vi "run.vi"(8 "error in (no error)":errorcluster, 11 "ImagingModeDL090130Frame in":refnum<class "ImagingModeDL090130Frame.lvclass">=refnum) -> (0 "error out":errorcluster, 3 "ImagingModeDL090130Frame out":refnum<class "ImagingModeDL090130Frame.lvclass">)   [LabVIEW 2010, in "ImagingModeDL090130Frame.lvclass"]
uses:
  ImagingModeDL090130Frame.lvclass
  internal_trigger_enum.ctl
  main/labview_source/controls/undock_button.ctl
  translation_mode_enum.ctl
  common/xcontrols/XSettings/XSettings/XSettings.xctl
  common/classes/GenericComponent/GenericComponent/GenericComponent.lvclass
  common/xcontrols/XIntensityCompensation/XIntensityCompensation/XIntensityCompensation.xctl
  speed_constant_enum.ctl
  control_refs.ctl
  state_enum.ctl
  common/classes/GenericToplevelComponent/GenericToplevelComponent/trigger_type_enum.ctl
  GenericImagingMode/GenericImagingMode/GenericImagingMode.lvclass
  ImagingModeDL090130Frame.lvclass/ImagingModeDL090130Frame.ctl
  Trajectory/GenericTrajectory/GenericTrajectory/GenericTrajectory.lvclass
  common/classes/ErrorController/ErrorController/class_data.vi
  common/classes/ErrorController/ErrorController/ErrorController.lvclass
panel:
  out "settings enforced?":bool
  in  "button:undock":T1
  in  "Tab Control":enum32{"User", "Debug", "About"}(tab)
  in  "XIntensityCompensation":cluster{"A":dbl, "lambda":dbl[unit], "C":dbl}(xcontrol)
  in  "translation mode":T2
  in  "return to origin?":bool=TRUE
  in  "step":dbl[unit] min=0.0 max=0.01 step=1e-07
  in  "no. of averagings":i32=1 caption="averaging" min=1 max=100
  in  "movie duration":dbl[unit]=10.24 min=0.0 max=3600.0
  in  "no. of frames":i32=20 caption="frames" min=1 max=100000
  in  "defineButton":bool
  in  "frame rate":dbl[unit]=1.953125 min=0.0 max=100.0
  in  "pixel dwell time":dbl[unit]=7.8125e-06 min=0.0 max=0.001
  in  "line scan time":dbl[unit]=0.002 min=0.0 max=1.0
  in  "y aspect":dbl=1.0 caption=":" min=0.0
  in  "x aspect":dbl=1.0 caption="aspect ratio (x:y)" min=0.0 step=1.0
  in  "y lines":i32=256 min=0 max=1000
  out "offset":dbl[unit]
  in  "x pixels":i32=256 min=0 max=1000 step=1
  out "frame no.":i32=12 caption="frame"
  out "repetition no.":i32=1 caption="repetition"
  in  "settings":refnum<class "GenericComponent.lvclass">(xcontrol)
  in  "keep constant":T3
  out "event handling loop counter":i32=10
  out "statemachine loop counter":i32=75
  out "event error":errorcluster
  out "action handler error":errorcluster
  out "finished?":bool
  out "last trigger":T4
  out "internal triggers":T4[](array[typedef])
  # "stack settings"
  # "frame settings"
  # "current values"
  # "ImagingModeDL090130Frame"
  # "Implemented by: \nDominik Langer, University of Zurich"
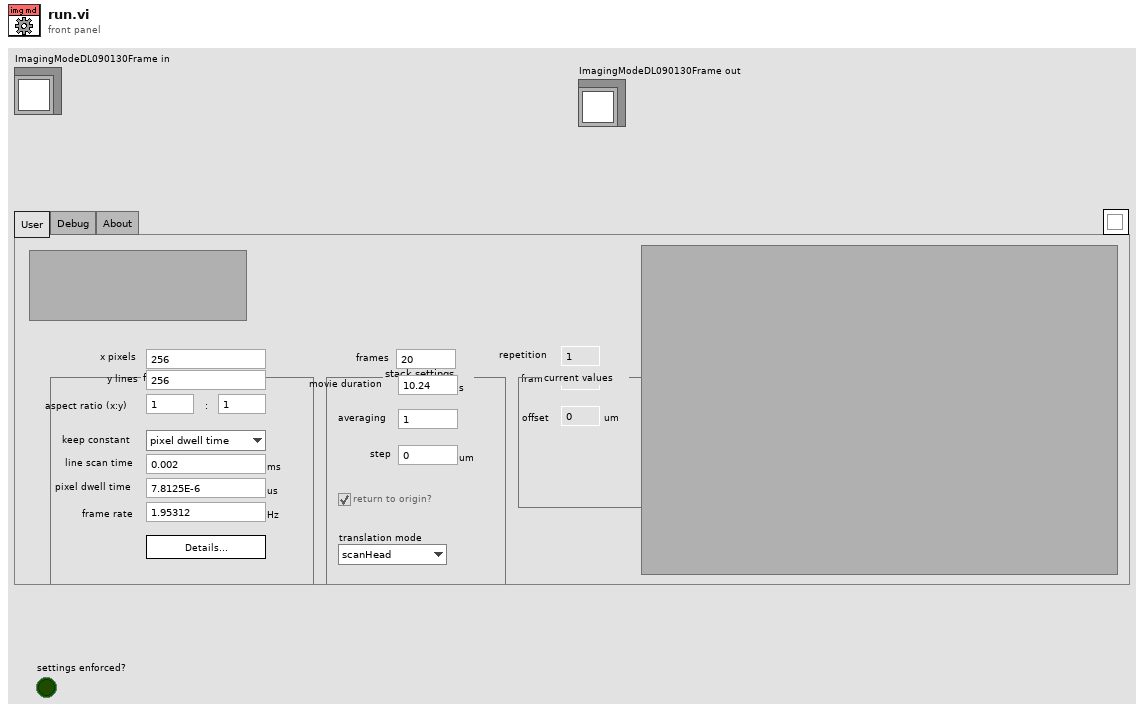
[diagram p1: front panel]
types:
  T1 = typedef "undock_button.ctl" = bool
  T2 = typedef "ImagingModeDL090130Frame.lvclass/translation_mode_enum.ctl" = enum16{"scanHead", "stage"}
  T3 = typedef "ImagingModeDL090130Frame.lvclass/speed_constant_enum.ctl" = enum16{"pixel dwell time", "line scan time", "frame rate"}
  T4 = typedef "ImagingModeDL090130Frame.lvclass/internal_trigger_enum.ctl" = enum16{"NULL", "initialise", "terminate", "start", "stop", "proceed", "update", "translate", "start scanning"}
  T5 = typedef "ImagingModeDL090130Frame.lvclass/control_refs.ctl" = cluster{"resolution controls":cluster{"x pixels":refnum<vi>, "y pixels":refnum<vi>, "ratio x factor":refnum<vi>, "ratio y factor":refnum<vi>}, "speed controls":cluster{"pixel dwell time":refnum<vi>, "line scan time":refnum<vi>, "frame rate":refnum<vi>, "keep constant":refnum<vi>}, "number of frames controls":cluster{"# of frames":refnum<vi>, "duration":refnum<vi>, "# of repetitions":refnum<vi>}, "current value indicators":cluster{"frame #":refnum<vi>, "repetition #":refnum<vi>, "offset":refnum<vi>}, "step controls":cluster{"step size":refnum<vi>, "return to origin?":refnum<vi>, "translation mode":refnum<vi>, "XIntensityCompensation":refnum<vi>}, "settings":refnum<vi>, "defineButton":refnum<vi>, "settings enforced?":refnum<vi>}
  T6 = typedef "ImagingModeDL090130Frame.lvclass/state_enum.ctl" = enum16{"idle", "sweep (scanning)", "sweep (translating)"}
  T7 = typedef "trigger_type_enum.ctl" = enum8{"external", "internal", "common"}
  T8 = typedef "main_trigger_enum.ctl" = enum16{"NULL", "initialise", "terminate", "start", "stop", "change objective", "change experimentController", "change imagingMode", "save notebook", "started saving", "finished saving", "expCtr ready", "expCtr missing", "imgMd ready", "imgMd missing", "scanHd ready", "scanHd missing", "DAQ ready", "DAQ missing", "imgAsm ready", "imgAsm missing", "dataColl ready", "dataColl missing", "display ready", "display missing", "analysr ready", "analysr missing", "instrmnt ready", "instrmnt missing", "stimltr ready", "stimltr missing", "stage ready", "stage missing"}
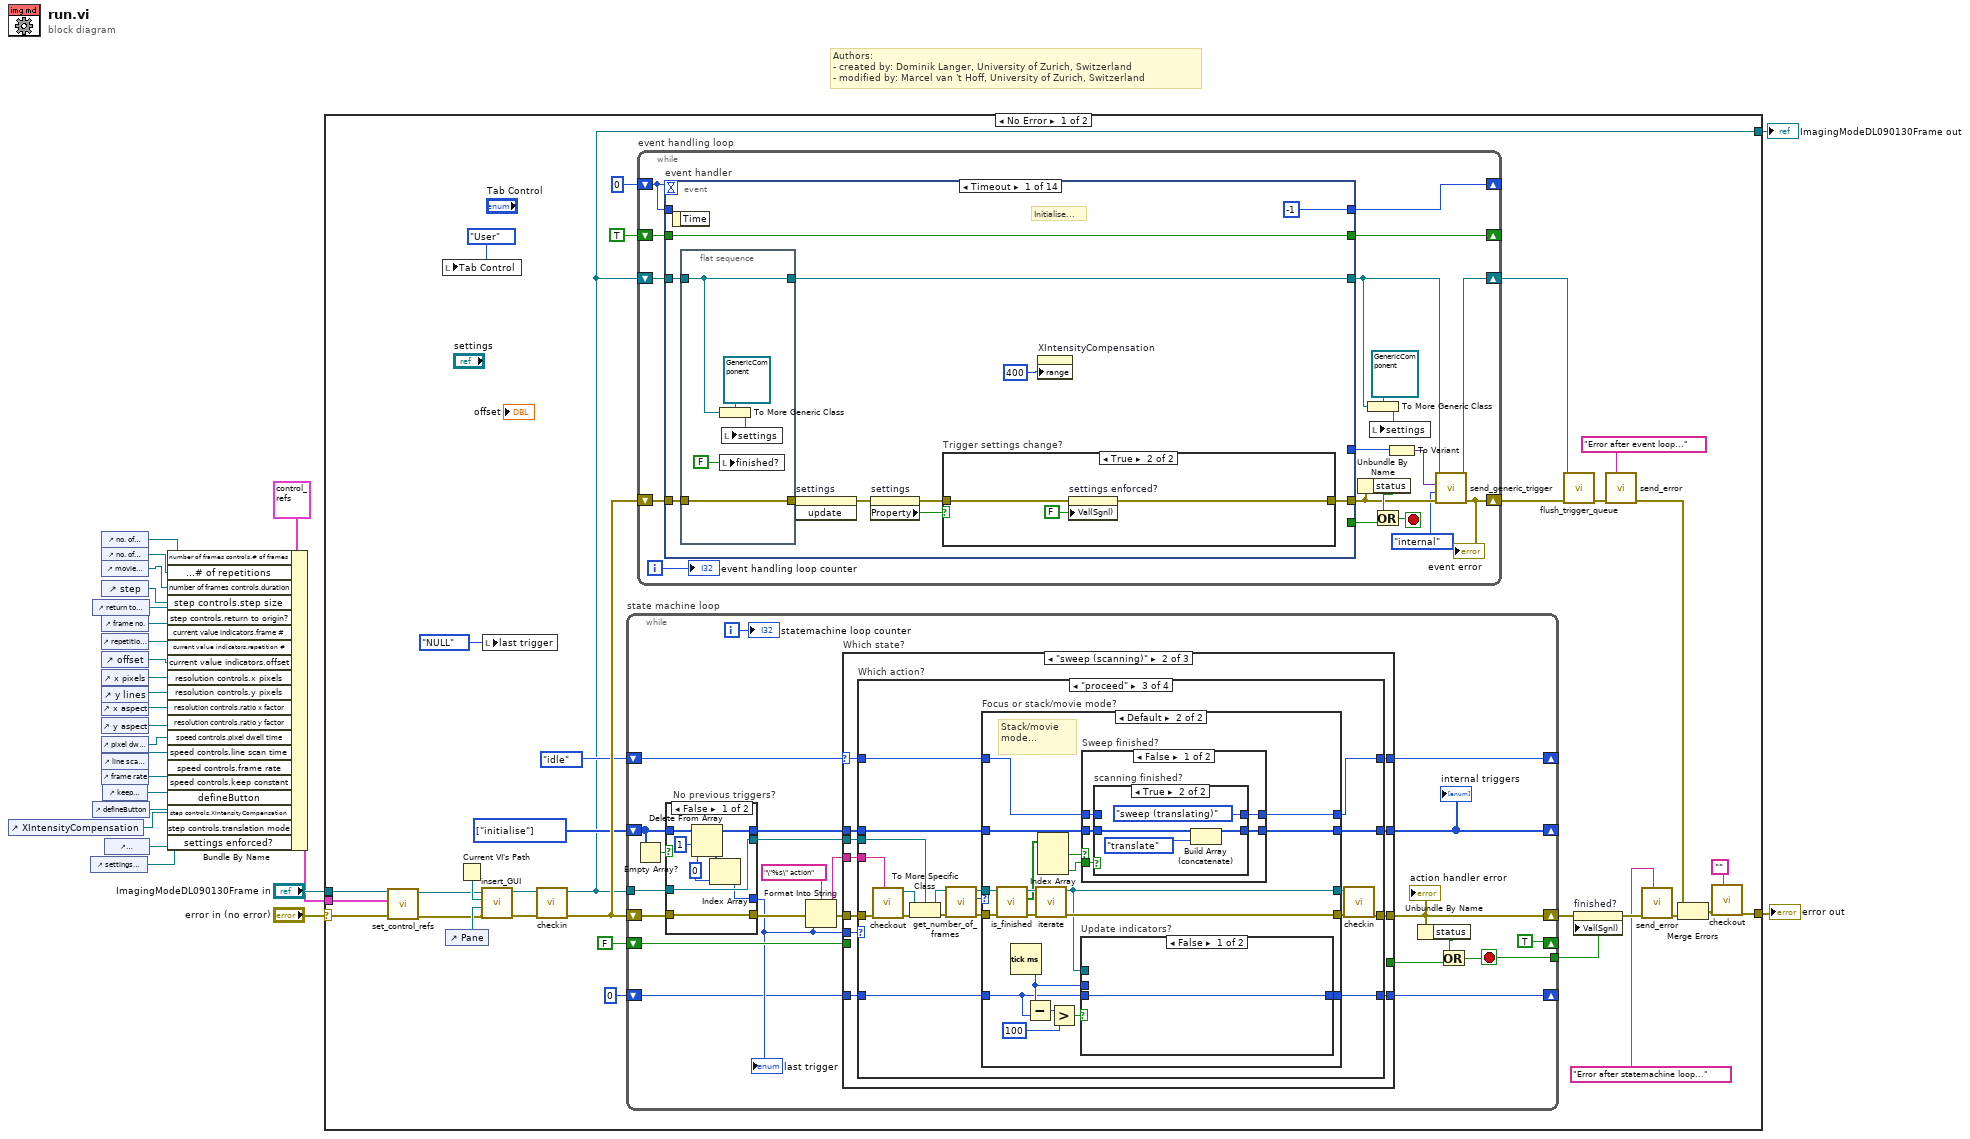
[diagram p0: block diagram]
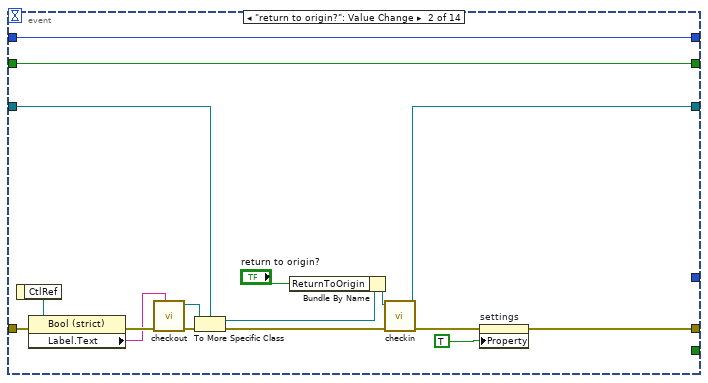
[diagram p3: hidden frame]
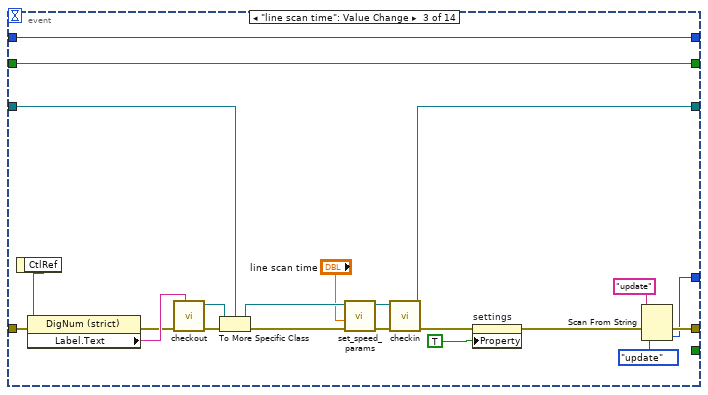
[diagram p4: hidden frame]
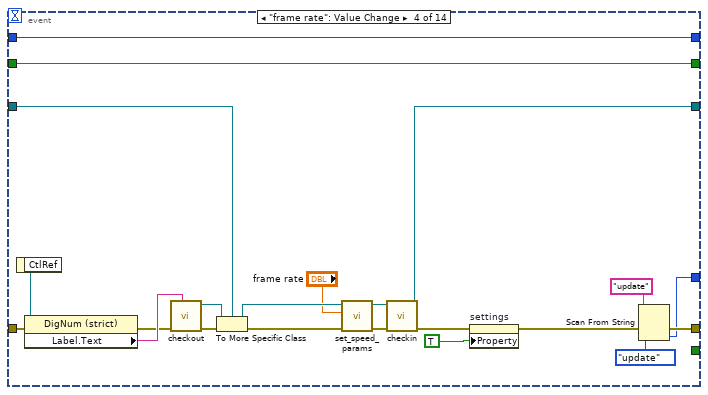
[diagram p5: hidden frame]
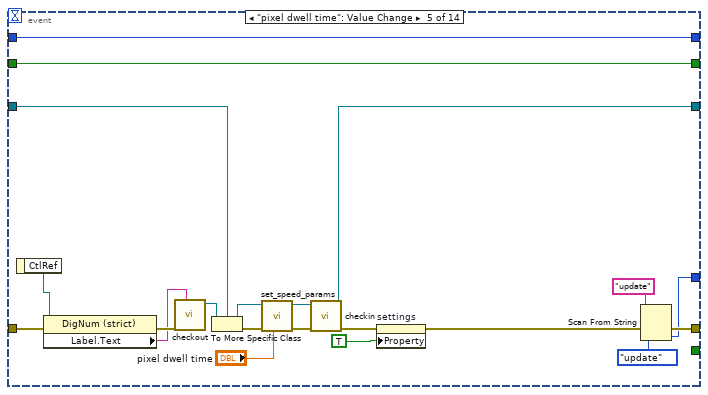
[diagram p6: hidden frame]
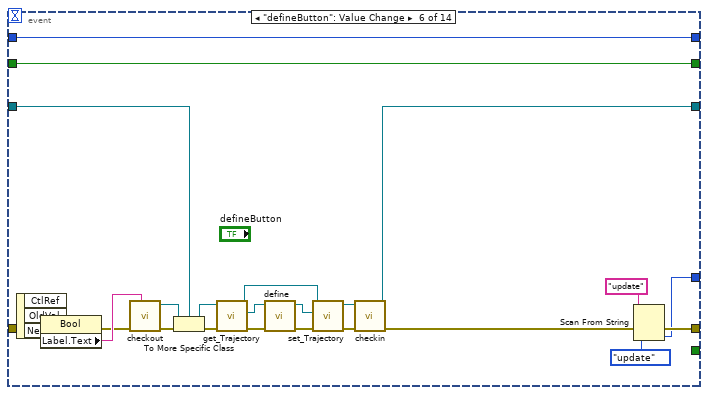
[diagram p7: hidden frame]
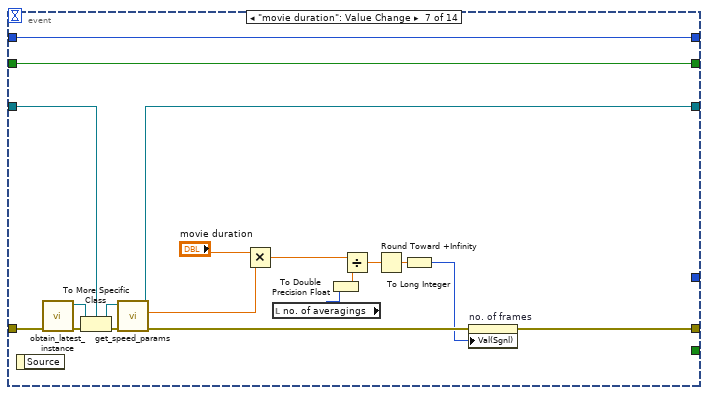
[diagram p8: hidden frame]
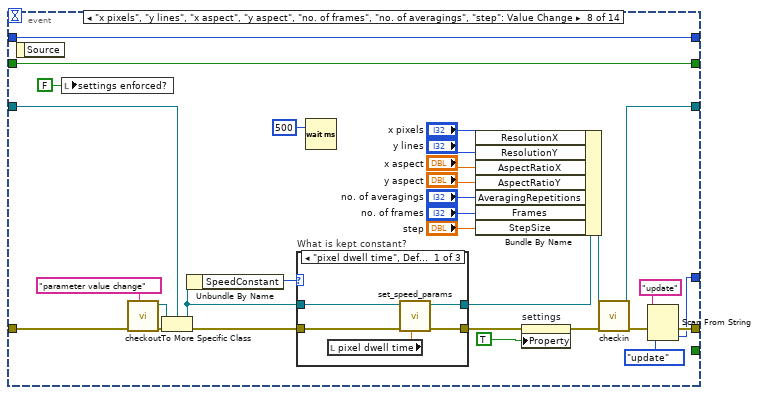
[diagram p9: hidden frame]
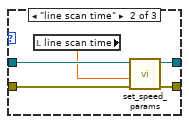
[diagram p10: hidden frame]
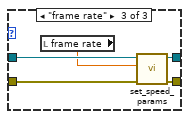
[diagram p11: hidden frame]
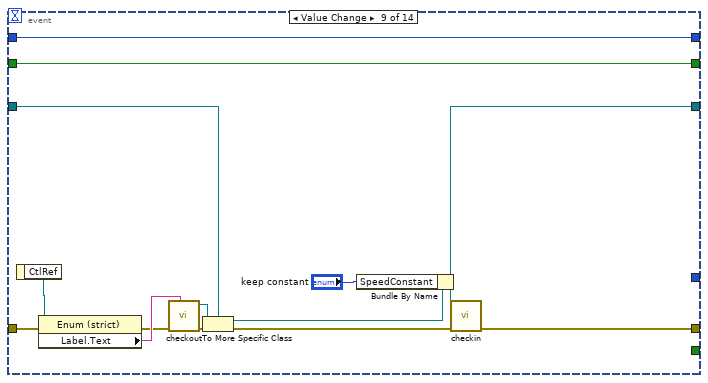
[diagram p12: hidden frame]
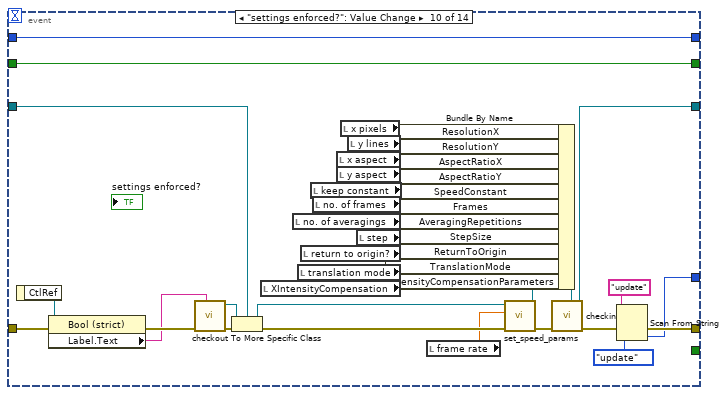
[diagram p13: hidden frame]
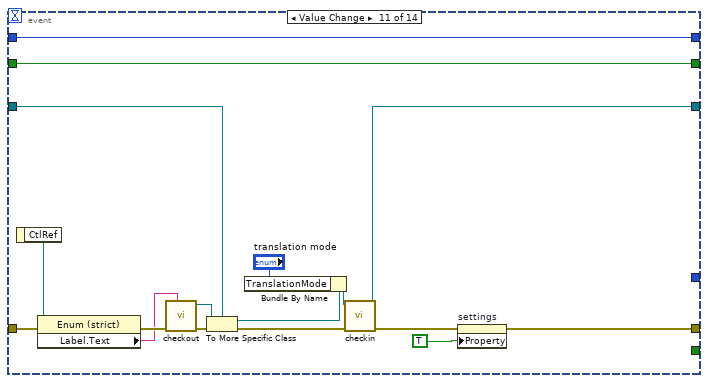
[diagram p14: hidden frame]
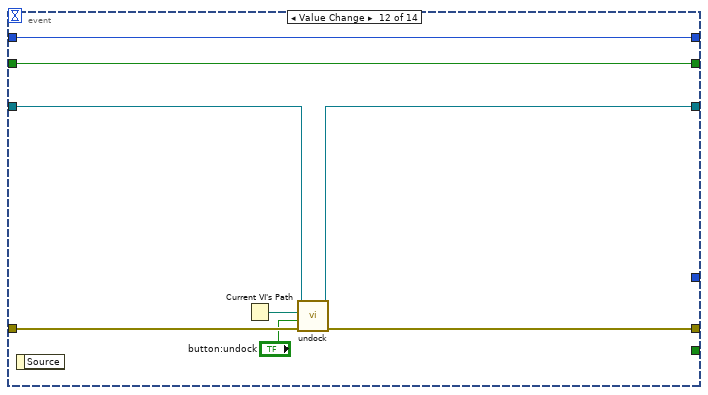
[diagram p15: hidden frame]
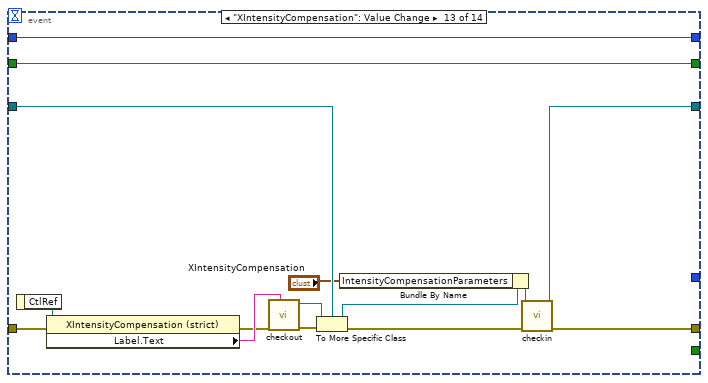
[diagram p16: hidden frame]
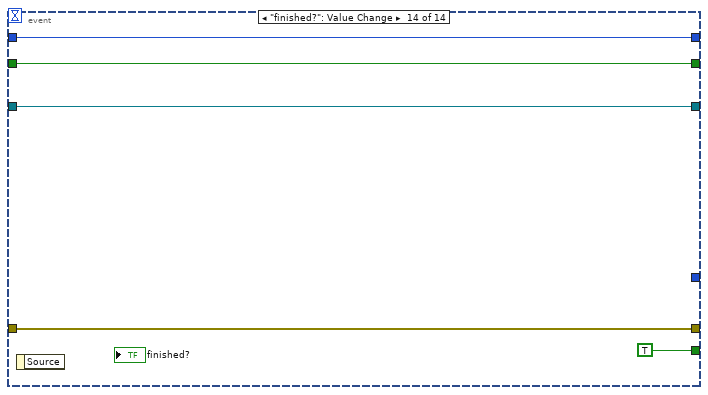
[diagram p17: hidden frame]
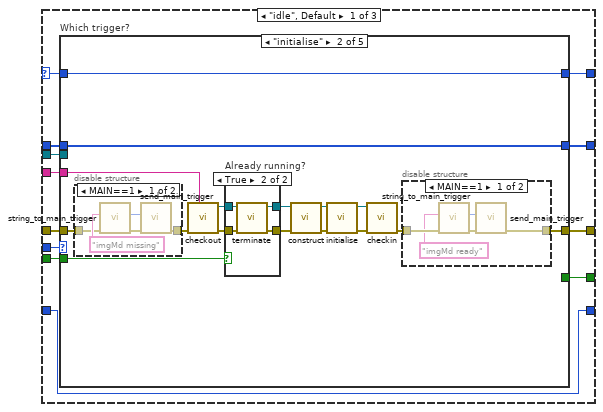
[diagram p18: hidden frame]
diagram:
  # "Authors: \n- created by: Dominik Langer, University of Zurich, Switzerland\n- modified by: Marcel van 't Hoff, University of Zurich, Switzerland"
  n1 = control-ref of="XIntensityCompensation"() -> (w4:refnum<vi>)
  n2 = control-ref of="settings enforced?"() -> (w2:refnum<vi>)
  n3 = control-ref of="return to origin?"() -> (w5:refnum<vi>)
  n4 = control-ref of="defineButton"() -> (w14:refnum<vi>)
  n5 = control-ref of="no. of frames"() -> (w10:refnum<vi>)
  n6 = control-ref of="no. of averagings"() -> (w8:refnum<vi>)
  n7 = control-ref of="movie duration"() -> (w9:refnum<vi>)
  n8 = control-ref of="step"() -> (w7:refnum<vi>)
  n9 = control-ref of="frame no."() -> (w21:refnum<vi>)
  n10 = control-ref of="repetition no."() -> (w22:refnum<vi>)
  n11 = control-ref of="offset"() -> (w24:refnum<vi>)
  n12 = control-ref of="x pixels"() -> (w23:refnum<vi>)
  n13 = control-ref of="y lines"() -> (w17:refnum<vi>)
  n14 = control-ref of="x aspect"() -> (w16:refnum<vi>)
  n15 = control-ref of="y aspect"() -> (w15:refnum<vi>)
  n16 = control-ref of="pixel dwell time"() -> (w11:refnum<vi>)
  n17 = control-ref of="line scan time"() -> (w12:refnum<vi>)
  n18 = control-ref of="frame rate"() -> (w13:refnum<vi>)
  n19 = control-ref of="keep constant"() -> (w1:refnum<vi>)
  n20 = control-ref of="translation mode"() -> (w6:refnum<vi>)
  n21 = Bundle By Name(cluster=T5 {"resolution controls"={"x pixels"=refnum, "y pixels"=refnum, "ratio x factor"=refnum, "ratio y factor"=refnum}, "speed controls"={"pixel dwell time"=refnum, "line scan time"=refnum, "frame rate"=refnum, "keep constant"=refnum}, "number of frames controls"={"# of frames"=refnum, "duration"=refnum, "# of repetitions"=refnum}, "current value indicators"={"frame #"=refnum, "repetition #"=refnum, "offset"=refnum}, "step controls"={"step size"=refnum, "return to origin?"=refnum, "translation mode"=refnum, "XIntensityCompensation"=refnum}, "settings"=refnum, "defineButton"=refnum, "settings enforced?"=refnum} ("control refs"), "number of frames controls.# of frames"=w10, "number of frames controls.# of repetitions"=w8, "number of frames controls.duration"=w9, "step controls.step size"=w7, "step controls.return to origin?"=w5, "current value indicators.frame #"=w21, "current value indicators.repetition #"=w22, "current value indicators.offset"=w24, "resolution controls.x pixels"=w23, "resolution controls.y pixels"=w17, "resolution controls.ratio x factor"=w16, "resolution controls.ratio y factor"=w15, "speed controls.pixel dwell time"=w11, "speed controls.line scan time"=w12, "speed controls.frame rate"=w13, "speed controls.keep constant"=w1, "defineButton"=w14, "step controls.XIntensityCompensation"=w4, "step controls.translation mode"=w6, "settings enforced?"=w2) -> (w18:T5)
  n22 = case shown="No Error" "error in (no error)" {
    selector: "error in (no error)" -> [w42 w632]
    tunnel: [w45 w632] -> w26
    tunnel: [w29 w631] -> w25
    tunnel: "ImagingModeDL090130Frame in" -> [w38 w631]
    tunnel: w18 -> [w39 _]
    frame No Error {
      w33 = T4[] [enum."initialise"] items=["NULL", "initialise", "terminate", "start", "stop", "proceed", "update", "translate", "start scanning"]
      n23 = call "set_control_refs.vi"("error in (no error)"=w42, "control refs"=w39, "ImagingModeDL090130Frame in"=w38) -> ("error out"=w40:errorcluster, "ImagingModeDL090130Frame out"=w41:refnum<class "ImagingModeDL090130Frame.lvclass">)  [unwired: 7 in]
      n24 = local write "Tab Control"(enum32{"User", "Debug", "About"}."User" ("Tab Control")) -> ()
      n25 = control-ref of="Pane"() -> (w51:refnum<vi>)
      n26 = Current VI's Path() -> (path=w53:path)
      n27 = call-dynamic "insert_GUI.vi"("error in (no error)"=w40, "Pane"=w51, "VI path"=w53, "GenericComponent in"=w41) -> ("error out"=w28:errorcluster, "GenericComponent out"=w37:refnum<class "ImagingModeDL090130Frame.lvclass">)  [unwired: 6 in]
      n28 = local write "last trigger"(internal_trigger_enum."NULL" ("last trigger")) -> ()
      n29 = call-dynamic "checkin.vi"("error in (no error)"=w28, "GenericScanMode in"=w37) -> ("error out"=w55:errorcluster, "GenericScanMode out"=w29:refnum<class "ImagingModeDL090130Frame.lvclass">)  [unwired: 8 in]
      n30 = while "state machine loop" {
        shift-right: [TRUE] -> _
        shift-left: FALSE -> [w369]
        tunnel: w29 -> [w380]
        tunnel: [w378] -> w36
        shift-right: [w375] -> w56
        shift-left: w55 -> [w379]
        shift-right: [w365] -> _
        shift-left: w33 -> [w367]
        shift-right: [w363] -> _
        shift-left: state_enum."idle" ("state") -> [w364]
        shift-right: [w359] -> _
        shift-left: u32 0 ("millisecond timer value") -> [w360]
        i -> [w361]
        stop <- w378 stop-if-true
        n31 = Empty Array?(array=w367) -> (empty?=w368:bool)
        n32 = case "No previous triggers?" shown="False" w368 {
          tunnel: w380 -> [w622 w630]
          tunnel: w379 -> [w624 w629]
          tunnel: [w622 w628] -> w377
          tunnel: [w617 w627] -> w362
          tunnel: [w624 w626] -> w373
          tunnel: w367 -> [w623 w625]
          tunnel: [w620 w625] -> w366
          frame False {
            w618 = 0 ("index")
            n33 = Delete From Array(array=w623, length=1, index=w618) -> (deleted portion=w619:T4[], array with subset deleted=w620:T4[])
            n34 = Index Array(array=w619, index=w618) -> (element=w617:T4)
          }
          frame True {
            n35 = call-dynamic "fetch_and_translate_trigger.vi"("error in (no error)"=w629, "ImagingModeDL090130Frame in"=w630) -> ("error out"=w626:errorcluster, "internal trigger"=w627:T4, "ImagingModeDL090130Frame out"=w628:refnum<class "ImagingModeDL090130Frame.lvclass">)  [unwired: 6 in, 1 out]
          }
        }
        "last trigger" <- w362
        n36 = Format Into String(format string="\"%s\" action", error in=w373, w362) -> (resulting string=w371:string, error out=w372:errorcluster)  [unwired: 1 in]
        n37 = case "Which state?" shown="\"sweep (scanning)\"" w364 {
          selector: w364 -> [w384 w478 w589]
          tunnel: w377 -> [w393 w481 w582]
          tunnel: [w392 _ _] -> w376
          tunnel: [w391 w483 w584] -> w375
          tunnel: w372 -> [w390 w484 w586]
          tunnel: w371 -> [w389 w480 w581]
          tunnel: w369 -> [w388 _ _]
          tunnel: w366 -> [w387 w482 w587]
          tunnel: w362 -> [w386 w476 w585]
          tunnel: [w385 w479 w583] -> w365
          tunnel: [w383 w477 w588] -> w363
          tunnel: w360 -> [w382 w475 w580]
          tunnel: [w382 w474 w580] -> w359
          frame "idle", Default {
            n38 = case "Which trigger?" shown="\"initialise\"" w386 {
              tunnel: w390 -> [w396 w398 w434 w455 w465]
              tunnel: w393 -> [_ _ _ w452 w463]
              tunnel: [w396 w400 w432 w454 w464] -> w391
              tunnel: [_ _ TRUE _ _] -> w392
              tunnel: w387 -> [w395 w412 w440 w451 w473]
              tunnel: [w395 w412 w440 w450 w473] -> w385
              tunnel: w389 -> [_ w409 w435 w453 w466]
              tunnel: w388 -> [_ w402 _ _ _]
              tunnel: [w394 w399 w431 state_enum."sweep (scanning)" ("state") w462] -> w383
              tunnel: w384 -> [w394 w399 w431 _ w462]
              frame "NULL", Default {
              }
              frame "initialise" {
                n39 = disable-structure shown="MAIN==1" {
                  disable-tunnel: w398 -> [w413 w418]
                  disable-tunnel: [w417 w418] -> w397
                  frame condition #0 {
                    n40 = call "string_to_main_trigger.vi"("error in (no error)"=w413, "trigger string"="imgMd missing") -> ("error out"=w416:errorcluster, "main trigger"=w415:T8)  [unwired: 8 in]
                    n41 = call "send_main_trigger.vi"("error in (no error)"=w416, "trigger"=w415) -> ("error out"=w417:errorcluster)  [unwired: 9 in]
                  }
                  frame condition #1 (active) {
                  }
                }
                n42 = call "checkout.vi"("locked by?"=w409, "error in (no error)"=w397) -> ("error out"=w406:errorcluster, "GenericScanMode out"=w405:refnum<class "GenericImagingMode.lvclass">)  [unwired: 8 in]
                n43 = case "Already running?" shown="True" w402 {
                  tunnel: w406 -> [w426 w430]
                  tunnel: w405 -> [w425 w429]
                  tunnel: [w425 w428] -> w404
                  tunnel: [w426 w427] -> w403
                  frame False {
                  }
                  frame True {
                    n44 = call-dynamic "terminate.vi"("error in (no error)"=w430, "GenericPlugin in"=w429) -> ("error out"=w427:errorcluster, "GenericPlugin out"=w428:refnum<class "GenericImagingMode.lvclass">)  [unwired: 8 out]
                  }
                }
                n45 = call-dynamic "construct.vi"("error in (no error)"=w403, "GenericPlugin in"=w404) -> ("error out"=w408:errorcluster, "GenericPlugin out"=w411:refnum<class "GenericImagingMode.lvclass">)  [unwired: 2 in, 6 out]
                n46 = call-dynamic "initialise.vi"("error in (no error)"=w408, "GenericPlugin in"=w411) -> ("error out"=w407:errorcluster, "GenericPlugin out"=w410:refnum<class "GenericImagingMode.lvclass">)  [unwired: 8 out]
                n47 = call-dynamic "checkin.vi"("error in (no error)"=w407, "GenericScanMode in"=w410) -> ("error out"=w401:errorcluster)  [unwired: 8 in, 1 out]
                n48 = disable-structure shown="MAIN==1" {
                  disable-tunnel: w401 -> [w422 w424]
                  disable-tunnel: [w423 w424] -> w400
                  frame condition #0 {
                    n49 = call "string_to_main_trigger.vi"("error in (no error)"=w422, "trigger string"="imgMd ready") -> ("error out"=w421:errorcluster, "main trigger"=w420:T8)  [unwired: 8 in]
                    n50 = call "send_main_trigger.vi"("error in (no error)"=w421, "trigger"=w420) -> ("error out"=w423:errorcluster)  [unwired: 9 in]
                  }
                  frame condition #1 (active) {
                  }
                }
              }
              frame "terminate" {
                n51 = disable-structure shown="MAIN==1" {
                  disable-tunnel: w434 -> [w445 w447]
                  disable-tunnel: [w446 w447] -> w433
                  frame condition #0 {
                    n52 = call "string_to_main_trigger.vi"("error in (no error)"=w445, "trigger string"="imgMd missing") -> ("error out"=w443:errorcluster, "main trigger"=w444:T8)  [unwired: 8 in]
                    n53 = call "send_main_trigger.vi"("error in (no error)"=w443, "trigger"=w444) -> ("error out"=w446:errorcluster)  [unwired: 9 in]
                  }
                  frame condition #1 (active) {
                  }
                }
                n54 = call "checkout.vi"("locked by?"=w435, "error in (no error)"=w433) -> ("error out"=w437:errorcluster, "GenericScanMode out"=w439:refnum<class "GenericImagingMode.lvclass">)  [unwired: 8 in]
                n55 = call-dynamic "terminate.vi"("error in (no error)"=w437, "GenericPlugin in"=w439) -> ("error out"=w436:errorcluster, "GenericPlugin out"=w438:refnum<class "GenericImagingMode.lvclass">)  [unwired: 8 out]
                n56 = call-dynamic "checkin.vi"("error in (no error)"=w436, "GenericScanMode in"=w438) -> ("error out"=w432:errorcluster)  [unwired: 8 in, 1 out]
              }
              frame "start" {
                n57 = call "checkout.vi"("locked by?"=w453, "error in (no error)"=w455) -> ("error out"=w456:errorcluster, "GenericScanMode out"=w457:refnum<class "GenericImagingMode.lvclass">)  [unwired: 8 in]
                n58 = To More Specific Class(target class=w452, reference=w457, error in=w456) -> (specific class reference=w460:refnum<class "ImagingModeDL090130Frame.lvclass">, error out=w461:errorcluster)
                n59 = call-dynamic "start_sweep.vi"("error in (no error)"=w461, "ImagingModeDL090130Frame in"=w460) -> ("error out"=w459:errorcluster, "ImagingModeDL090130Frame out"=w458:refnum<class "ImagingModeDL090130Frame.lvclass">)  [unwired: 8 out]
                n60 = call-dynamic "checkin.vi"("error in (no error)"=w459, "GenericScanMode in"=w458) -> ("error out"=w454:errorcluster)  [unwired: 8 in, 1 out]
                n61 = Build Array (concatenate)(w451, internal_trigger_enum."start scanning" ("internal trigger")) -> (w450:T4[])
              }
              frame "update" {
                n62 = call "checkout.vi"("locked by?"=w466, "error in (no error)"=w465) -> ("error out"=w467:errorcluster, "GenericScanMode out"=w468:refnum<class "GenericImagingMode.lvclass">)  [unwired: 8 in]
                n63 = To More Specific Class(target class=w463, reference=w468, error in=w467) -> (specific class reference=w472:refnum<class "ImagingModeDL090130Frame.lvclass">, error out=w469:errorcluster)
                n64 = call-dynamic "update.vi"("error in (no error)"=w469, "ImagingModeDL090130Frame in"=w472) -> ("error out"=w470:errorcluster, "ImagingModeDL090130Frame out"=w471:refnum<class "ImagingModeDL090130Frame.lvclass">)  [unwired: 8 out]
                n65 = call-dynamic "checkin.vi"("error in (no error)"=w470, "GenericScanMode in"=w471) -> ("error out"=w464:errorcluster)  [unwired: 8 in, 1 out]
              }
            }
          }
          frame "sweep (scanning)" {
            n66 = case "Which action?" shown="\"proceed\"" w476 {
              tunnel: w484 -> [w488 w502 w512 w570]
              tunnel: w481 -> [_ w503 w513 w572]
              tunnel: [w488 w501 w511 w569] -> w483
              tunnel: w482 -> [w487 w499 w509 w579]
              tunnel: [w487 w499 w508 w579] -> w479
              tunnel: w480 -> [_ w500 w510 w571]
              tunnel: w478 -> [w486 _ w507 w568]
              tunnel: [w486 state_enum."idle" ("state") w506 w568] -> w477
              tunnel: w475 -> [w485 w489 w505 w567]
              tunnel: [w485 w489 w504 w567] -> w474
              frame "NULL", Default {
              }
              frame "stop" {
                n67 = call "checkout.vi"("locked by?"=w500, "error in (no error)"=w502) -> ("error out"=w496:errorcluster, "GenericScanMode out"=w497:refnum<class "GenericImagingMode.lvclass">)  [unwired: 8 in]
                n68 = To More Specific Class(target class=w503, reference=w497, error in=w496) -> (specific class reference=w494:refnum<class "ImagingModeDL090130Frame.lvclass">, error out=w492:errorcluster)
                n69 = call-dynamic "stop_scanning.vi"("error in (no error)"=w492, "ScanModeDL090923Scaffold in"=w494) -> ("error out"=w491:errorcluster, "ScanModeDL090923Scaffold out"=w493:refnum<class "ImagingModeDL090130Frame.lvclass">)  [unwired: 8 out]
                n70 = call-dynamic "stop_sweep.vi"("error in (no error)"=w491, "ImagingModeDL090130Frame in"=w493) -> ("error out"=w495:errorcluster, "ImagingModeDL090130Frame out"=w498:refnum<class "ImagingModeDL090130Frame.lvclass">)  [unwired: 8 in]
                n71 = call-dynamic "checkin.vi"("error in (no error)"=w495, "GenericScanMode in"=w498) -> ("error out"=w501:errorcluster)  [unwired: 8 in, 1 out]
              }
              frame "proceed" {
                n72 = call "checkout.vi"("locked by?"=w510, "error in (no error)"=w512) -> ("error out"=w514:errorcluster, "GenericScanMode out"=w515:refnum<class "GenericImagingMode.lvclass">)  [unwired: 8 in]
                n73 = To More Specific Class(target class=w513, reference=w515, error in=w514) -> (specific class reference=w516:refnum<class "ImagingModeDL090130Frame.lvclass">, error out=w517:errorcluster)
                n74 = call-dynamic "get_number_of_frames.vi"("error in (no error)"=w517, "ImagingModeDL090130Frame in"=w516) -> ("error out"=w519:errorcluster, "number of frames"=w518:i32, "ImagingModeDL090130Frame out"=w520:refnum<class "ImagingModeDL090130Frame.lvclass">)  [unwired: 7 out]
                n75 = case "Focus or stack/movie mode?" shown="Default" w518 {
                  tunnel: [w527 w540] -> w521
                  tunnel: w509 -> [w526 w546]
                  tunnel: [w526 w545] -> w508
                  tunnel: w519 -> [w527 w542]
                  tunnel: w520 -> [w525 w541]
                  tunnel: [w525 w534] -> w522
                  tunnel: w507 -> [w524 w539]
                  tunnel: [w524 w538] -> w506
                  tunnel: w505 -> [w523 w531]
                  tunnel: [w523 w533] -> w504
                  frame -1 {
                    # "Focus mode: don't react..."
                  }
                  frame Default {
                    # "Stack/movie mode..."
                    n76 = call-dynamic "is_finished.vi"("error in (no error)"=w542, "ImagingModeDL090130Frame in"=w541) -> ("error out"=w544:errorcluster, "finished?"=w537:bool[], "ImagingModeDL090130Frame out"=w543:refnum<class "ImagingModeDL090130Frame.lvclass">)  [unwired: 7 out]
                    n77 = Tick Count (ms)() -> (millisecond timer value=w532:u32)
                    n78 = Subtract(x=w532, y=w531) -> (x-y=w529:u32)
                    n79 = call-dynamic "iterate.vi"("error in (no error)"=w544, "ImagingModeDL090130Frame in"=w543) -> ("error out"=w540:errorcluster, "ImagingModeDL090130Frame out"=w534:refnum<class "ImagingModeDL090130Frame.lvclass">)  [unwired: 8 out]
                    n80 = Index Array(array=w537) -> (element #1=w536:bool, element #3=w535:bool)  [unwired: 3 in, 1 out]
                    n81 = Greater?(x=w529, y=u32 100) -> (0:w530:bool)
                    n82 = case "Update indicators?" shown="False" w530 {
                      tunnel: w534 -> [_ w551]
                      tunnel: [w547 w548] -> w533
                      tunnel: w531 -> [w547 _]
                      tunnel: w532 -> [_ w548]
                      frame False {
                      }
                      frame True {
                        # "Strangely, if they are updated to often, it, it gets slowed down..."
                        n83 = Unbundle By Name(w551) -> ("current frame"=→"frame no.":i32, "current repetition"=→"repetition no.":i32)
                      }
                    }
                    n84 = case "Sweep finished?" shown="False" w536 {
                      tunnel: w546 -> [w556 w565]
                      tunnel: w535 -> [w552 _]
                      tunnel: [w555 w564] -> w545
                      tunnel: w539 -> [w554 w563]
                      tunnel: [w553 w563] -> w538
                      frame False {
                        n85 = case "scanning finished?" shown="True" w552 {
                          tunnel: w556 -> [w558 w562]
                          tunnel: [w558 w561] -> w555
                          tunnel: w554 -> [w557 _]
                          tunnel: [w557 state_enum."sweep (translating)" ("state")] -> w553
                          frame False {
                          }
                          frame True {
                            n86 = Build Array (concatenate)(w562, internal_trigger_enum."translate" ("internal trigger")) -> (w561:T4[])
                          }
                        }
                      }
                      frame True {
                        n87 = Build Array (concatenate)(w565, internal_trigger_enum."stop" ("internal trigger")) -> (w564:T4[])
                      }
                    }
                  }
                }
                n88 = call-dynamic "checkin.vi"("error in (no error)"=w521, "GenericScanMode in"=w522) -> ("error out"=w511:errorcluster)  [unwired: 8 in, 1 out]
              }
              frame "start scanning" {
                n89 = call "checkout.vi"("locked by?"=w571, "error in (no error)"=w570) -> ("error out"=w573:errorcluster, "GenericScanMode out"=w574:refnum<class "GenericImagingMode.lvclass">)  [unwired: 8 in]
                n90 = To More Specific Class(target class=w572, reference=w574, error in=w573) -> (specific class reference=w576:refnum<class "ImagingModeDL090130Frame.lvclass">, error out=w575:errorcluster)
                n91 = call-dynamic "start_scanning.vi"("error in (no error)"=w575, "ScanModeDL090923Scaffold in"=w576) -> ("error out"=w577:errorcluster, "ScanModeDL090923Scaffold out"=w578:refnum<class "ImagingModeDL090130Frame.lvclass">)  [unwired: 8 out]
                n92 = call-dynamic "checkin.vi"("error in (no error)"=w577, "GenericScanMode in"=w578) -> ("error out"=w569:errorcluster)  [unwired: 8 in, 1 out]
              }
            }
          }
          frame "sweep (translating)" {
            n93 = case "Which action?" shown="\"translate\"" w585 {
              tunnel: w586 -> [w590 w597 w602 w610]
              tunnel: w582 -> [_ _ _ w609]
              tunnel: [w590 w597 w602 w608] -> w584
              tunnel: w587 -> [w592 w594 w600 w616]
              tunnel: [w592 w595 w599 w616] -> w583
              tunnel: w581 -> [_ _ _ w611]
              tunnel: w589 -> [w591 _ _ w607]
              tunnel: [w591 state_enum."sweep (scanning)" ("state") state_enum."sweep (scanning)" ("state") w607] -> w588
              frame "NULL", Default {
              }
              frame "stop" {
                n94 = Build Array (concatenate)(internal_trigger_enum."stop" ("internal trigger"), w594) -> (w595:T4[])
              }
              frame "proceed" {
                n95 = Build Array (concatenate)(w600, internal_trigger_enum."start scanning" ("internal trigger")) -> (w599:T4[])
              }
              frame "translate" {
                n96 = call "checkout.vi"("locked by?"=w611, "error in (no error)"=w610) -> ("error out"=w612:errorcluster, "GenericScanMode out"=w613:refnum<class "GenericImagingMode.lvclass">)  [unwired: 8 in]
                n97 = To More Specific Class(target class=w609, reference=w613, error in=w612) -> (specific class reference=w606:refnum<class "ImagingModeDL090130Frame.lvclass">, error out=w605:errorcluster)
                n98 = call-dynamic "stop_scanning.vi"("error in (no error)"=w605, "ScanModeDL090923Scaffold in"=w606) -> ("error out"=w604:errorcluster, "ScanModeDL090923Scaffold out"=w603:refnum<class "ImagingModeDL090130Frame.lvclass">)  [unwired: 8 out]
                n99 = call-dynamic "translate.vi"("error in (no error)"=w604, "ImagingModeDL090130Frame in"=w603) -> ("error out"=w614:errorcluster, "ImagingModeDL090130Frame out"=w615:refnum<class "ImagingModeDL090130Frame.lvclass">)  [unwired: 8 out]
                n100 = call-dynamic "checkin.vi"("error in (no error)"=w614, "GenericScanMode in"=w615) -> ("error out"=w608:errorcluster)  [unwired: 8 in, 1 out]
              }
            }
          }
        }
        "action handler error" <- w375
        "internal triggers" <- w365
        n101 = Unbundle By Name(w375) -> ("status"=w374:bool)
        n102 = Or(x=w374, y=w376) -> (x .or. y?=w378:bool)
        "statemachine loop counter" <- w361
      }
      n103 = while "event handling loop" {
        shift-right: [w76] -> _
        shift-left: 0 -> [w77]
        shift-right: [w72] -> _
        shift-left: TRUE -> [w73]
        shift-right: [w67] -> w35
        shift-left: w55 -> [w75]
        shift-right: [w60] -> w30
        shift-left: w29 -> [w61]
        i -> [w74]
        stop <- w69 stop-if-true
        n104 = event "event handler" shown="[0] Timeout" {
          selector: _ -> [_ _ _ _ _ _ _ _ _ _ _ _ _ _]
          dyn-events: _ -> [_ _ _ _ _ _ _ _ _ _ _ _ _ _]
          timeout: w77 -> [_ _ _ _ _ _ _ _ _ _ _ _ _ _]
          tunnel: [-1 w114 w136 w158 w179 w203 w222 w252 w281 w313 w330 w338 w353 w358] -> w76
          tunnel: w77 -> [_ w114 w136 w158 w179 w203 w222 w252 w281 w313 w330 w338 w353 w358]
          tunnel: w75 -> [w87 w105 w126 w145 w170 w190 w221 w231 w269 w286 w320 w336 w342 w357]
          tunnel: [w79 w99 w120 w144 w164 w181 w205 w240 w273 w294 w314 w335 w348 w357] -> w68
          tunnel: [_ _ _ _ _ _ _ _ _ _ _ _ _ TRUE] -> w70
          tunnel: w73 -> [w86 w108 w135 w157 w178 w202 w214 w246 w280 w312 w329 w337 w352 w355]
          tunnel: [w86 w108 w135 w157 w178 w202 w214 w246 w280 w312 w329 w337 w352 w355] -> w72
          tunnel: [_ _ w119 w141 w163 w180 _ w239 _ w293 _ _ _ _] -> w64
          tunnel: [w84 w103 w124 w137 w172 w186 w213 w245 w270 w283 w319 w331 w345 w354] -> w59
          tunnel: w61 -> [w85 w102 w123 w140 w167 w185 w212 w244 w275 w309 w318 w332 w344 w354]
          event Timeout {
            # "Initialise..."
            n105 = event-data() -> ()  [unwired: 2 out]
            n106 = flat-sequence {
              tunnel: w87 -> [w93]
              tunnel: w85 -> [w94]
              tunnel: [w94] -> w84
              tunnel: [w93] -> w83
              frame #0 {
                n107 = To More Generic Class(target class=refnum<class "GenericComponent.lvclass"> refnum ("GenericComponent.lvclass"), reference=w94) -> (generic class reference=w96:refnum<class "GenericComponent.lvclass">)
                n108 = local write "finished?"(FALSE ("finished?")) -> ()
                n109 = local write "settings"(w96) -> ()
              }
            }
            n110 = invoke on="settings" class="XSettings (strict)" method="update"(error in=w83) -> (error out=w82:errorcluster)  [unwired: 2 in, 2 out]
            n111 = property on="settings" class="XSettings (strict)"(error in=w82) -> (error out=w80:errorcluster, "Property"=w81:bool)  [unwired: 1 in, 1 out]
            n112 = case "Trigger settings change?" shown="True" w81 {
              tunnel: w80 -> [w89 w92]
              tunnel: [w89 w90] -> w79
              frame False {
              }
              frame True {
                n113 = property on="settings enforced?" class="Bool (strict)"(error in=w92, "Val(Sgnl)"=FALSE ("Value (Signaling)")) -> (error out=w90:errorcluster)  [unwired: 1 in, 1 out]
              }
            }
            n114 = property on="XIntensityCompensation" class="XIntensityCompensation (strict)"("range"=400) -> ()  [unwired: 2 in, 2 out]
          }
          event "return to origin?": Value Change {
            n115 = event-data() -> ("CtlRef"=w107:refnum<vi>)  [unwired: 1 out]
            n116 = property class="Bool (strict)"(reference=w107, error in=w105) -> (error out=w106:errorcluster, "Label.Text"=w104:string)  [unwired: 1 out]
            n117 = call "checkout.vi"("locked by?"=w104, "error in (no error)"=w106) -> ("error out"=w113:errorcluster, "GenericScanMode out"=w112:refnum<class "GenericImagingMode.lvclass">)  [unwired: 8 in]
            n118 = To More Specific Class(target class=w102, reference=w112, error in=w113) -> (specific class reference=w110:refnum<class "ImagingModeDL090130Frame.lvclass">, error out=w111:errorcluster)
            n119 = Bundle By Name(cluster=w110, "ReturnToOrigin"="return to origin?") -> (w109:refnum<class "ImagingModeDL090130Frame.lvclass">)
            n120 = call-dynamic "checkin.vi"("error in (no error)"=w111, "GenericScanMode in"=w109) -> ("error out"=w100:errorcluster, "GenericScanMode out"=w103:refnum<class "ImagingModeDL090130Frame.lvclass">)  [unwired: 8 in]
            n121 = property on="settings" class="XSettings (strict)"(error in=w100, "Property"=TRUE ("is user-defined?")) -> (error out=w99:errorcluster)  [unwired: 1 in, 1 out]
          }
          event "line scan time": Value Change {
            n122 = event-data() -> ("CtlRef"=w127:refnum<vi>)  [unwired: 1 out]
            n123 = property class="DigNum (strict)"(reference=w127, error in=w126) -> (error out=w125:errorcluster, "Label.Text"=w128:string)  [unwired: 1 out]
            n124 = call "checkout.vi"("locked by?"=w128, "error in (no error)"=w125) -> ("error out"=w130:errorcluster, "GenericScanMode out"=w129:refnum<class "GenericImagingMode.lvclass">)  [unwired: 8 in]
            n125 = To More Specific Class(target class=w123, reference=w129, error in=w130) -> (specific class reference=w133:refnum<class "ImagingModeDL090130Frame.lvclass">, error out=w134:errorcluster)
            n126 = call-dynamic "set_speed_params.vi"("error in (no error)"=w134, "line-scan time"="line scan time", "ImagingModeDL090130Frame in"=w133) -> ("error out"=w131:errorcluster, "ImagingModeDL090130Frame out"=w132:refnum<class "ImagingModeDL090130Frame.lvclass">)  [unwired: 7 in]
            n127 = call-dynamic "checkin.vi"("error in (no error)"=w131, "GenericScanMode in"=w132) -> ("error out"=w116:errorcluster, "GenericScanMode out"=w124:refnum<class "ImagingModeDL090130Frame.lvclass">)  [unwired: 8 in]
            n128 = property on="settings" class="XSettings (strict)"(error in=w116, "Property"=TRUE ("is user-defined?")) -> (error out=w115:errorcluster)  [unwired: 1 in, 1 out]
            n129 = Scan From String(input string="update", error in=w115, default 1=internal_trigger_enum."update" ("internal trigger")) -> (error out=w120:errorcluster, output 1=w119:T4)  [unwired: 2 in, 2 out]
          }
          event "frame rate": Value Change {
            n130 = event-data() -> ("CtlRef"=w139:refnum<vi>)  [unwired: 1 out]
            n131 = property class="DigNum (strict)"(reference=w139, error in=w145) -> (error out=w149:errorcluster, "Label.Text"=w150:string)  [unwired: 1 out]
            n132 = call "checkout.vi"("locked by?"=w150, "error in (no error)"=w149) -> ("error out"=w152:errorcluster, "GenericScanMode out"=w151:refnum<class "GenericImagingMode.lvclass">)  [unwired: 8 in]
            n133 = To More Specific Class(target class=w140, reference=w151, error in=w152) -> (specific class reference=w155:refnum<class "ImagingModeDL090130Frame.lvclass">, error out=w156:errorcluster)
            n134 = call-dynamic "set_speed_params.vi"("error in (no error)"=w156, "frame rate"="frame rate", "ImagingModeDL090130Frame in"=w155) -> ("error out"=w153:errorcluster, "ImagingModeDL090130Frame out"=w154:refnum<class "ImagingModeDL090130Frame.lvclass">)  [unwired: 7 in]
            n135 = call-dynamic "checkin.vi"("error in (no error)"=w153, "GenericScanMode in"=w154) -> ("error out"=w147:errorcluster, "GenericScanMode out"=w137:refnum<class "ImagingModeDL090130Frame.lvclass">)  [unwired: 8 in]
            n136 = property on="settings" class="XSettings (strict)"(error in=w147, "Property"=TRUE ("is user-defined?")) -> (error out=w146:errorcluster)  [unwired: 1 in, 1 out]
            n137 = Scan From String(input string="update", error in=w146, default 1=internal_trigger_enum."update" ("internal trigger")) -> (error out=w144:errorcluster, output 1=w141:T4)  [unwired: 2 in, 2 out]
          }
          event "pixel dwell time": Value Change {
            n138 = event-data() -> ("CtlRef"=w171:refnum<vi>)  [unwired: 1 out]
            n139 = property class="DigNum (strict)"(reference=w171, error in=w170) -> (error out=w169:errorcluster, "Label.Text"=w168:string)  [unwired: 1 out]
            n140 = call "checkout.vi"("locked by?"=w168, "error in (no error)"=w169) -> ("GenericScanMode out"=w173:refnum<class "GenericImagingMode.lvclass">)  [unwired: 8 in, 1 out]
            n141 = To More Specific Class(target class=w167, reference=w173) -> (specific class reference=w176:refnum<class "ImagingModeDL090130Frame.lvclass">, error out=w177:errorcluster)  [unwired: 1 in]
            n142 = call-dynamic "set_speed_params.vi"("pixel-dwell time"="pixel dwell time", "error in (no error)"=w177, "ImagingModeDL090130Frame in"=w176) -> ("error out"=w174:errorcluster, "ImagingModeDL090130Frame out"=w175:refnum<class "ImagingModeDL090130Frame.lvclass">)  [unwired: 7 in]
            n143 = call-dynamic "checkin.vi"("error in (no error)"=w174, "GenericScanMode in"=w175) -> ("error out"=w160:errorcluster, "GenericScanMode out"=w172:refnum<class "ImagingModeDL090130Frame.lvclass">)  [unwired: 8 in]
            n144 = property on="settings" class="XSettings (strict)"(error in=w160, "Property"=TRUE ("is user-defined?")) -> (error out=w159:errorcluster)  [unwired: 1 in, 1 out]
            n145 = Scan From String(input string="update", error in=w159, default 1=internal_trigger_enum."update" ("internal trigger")) -> (error out=w164:errorcluster, output 1=w163:T4)  [unwired: 2 in, 2 out]
          }
          event "defineButton": Value Change {
            n146 = event-data() -> ("CtlRef"=w189:refnum<vi>)  [unwired: 3 out]
            n147 = property class="Bool"(reference=w189, error in=w190) -> (error out=w187:errorcluster, "Label.Text"=w188:string)  [unwired: 1 out]
            n148 = call "checkout.vi"("locked by?"=w188, "error in (no error)"=w187) -> ("error out"=w200:errorcluster, "GenericScanMode out"=w201:refnum<class "GenericImagingMode.lvclass">)  [unwired: 8 in]
            n149 = To More Specific Class(target class=w185, reference=w201, error in=w200) -> (specific class reference=w198:refnum<class "ImagingModeDL090130Frame.lvclass">, error out=w199:errorcluster)
            n150 = call-dynamic "get_Trajectory.vi"("error in (no error)"=w199, "ScanModeDL090923Scaffold in"=w198) -> ("error out"=w197:errorcluster, "Trajectory"=w196:refnum<class "GenericTrajectory.lvclass">, "ScanModeDL090923Scaffold out"=w191:refnum<class "ImagingModeDL090130Frame.lvclass">)  [unwired: 2 in, 5 out]
            n151 = call-dynamic "define.vi"("error in (no error)"=w197, "GenericTrajectory in"=w196) -> ("error out"=w195:errorcluster, "GenericTrajectory out"=w194:refnum<class "GenericTrajectory.lvclass">)  [unwired: 8 in]
            n152 = call-dynamic "set_Trajectory.vi"("error in (no error)"=w195, "GenericTrajectory.lvclass"=w194, "ScanModeDL090923Scaffold in"=w191) -> ("error out"=w193:errorcluster, "ScanModeDL090923Scaffold out"=w192:refnum<class "ImagingModeDL090130Frame.lvclass">)  [unwired: 7 in]
            n153 = call-dynamic "checkin.vi"("error in (no error)"=w193, "GenericScanMode in"=w192) -> ("error out"=w182:errorcluster, "GenericScanMode out"=w186:refnum<class "ImagingModeDL090130Frame.lvclass">)  [unwired: 8 in]
            n154 = Scan From String(input string="update", error in=w182, default 1=internal_trigger_enum."update" ("internal trigger")) -> (error out=w181:errorcluster, output 1=w180:T4)  [unwired: 2 in, 2 out]
          }
          event "movie duration": Value Change {
            n155 = event-data() -> ()  [unwired: 2 out]
            n156 = call "obtain_latest_instance.vi"("error in (no error)"=w221) -> ("error out"=w220:errorcluster, "GenericScanMode out"=w218:refnum<class "GenericImagingMode.lvclass">)  [unwired: 9 in]
            n157 = To More Specific Class(target class=w212, reference=w218, error in=w220) -> (specific class reference=w217:refnum<class "ImagingModeDL090130Frame.lvclass">, error out=w219:errorcluster)
            n158 = call-dynamic "get_speed_params.vi"("error in (no error)"=w219, "ImagingModeDL090130Frame in"=w217) -> ("error out"=w207:errorcluster, "frame rate"=w216:dbl[unit], "ImagingModeDL090130Frame out"=w213:refnum<class "ImagingModeDL090130Frame.lvclass">)  [unwired: 4 in, 3 out]
            n159 = Multiply(x="movie duration", y=w216) -> (x*y=w211:dbl)
            n160 = local read "no. of averagings"() -> (w204:i32)
            n161 = To Double Precision Float(number=w204) -> (double precision float=w209:dbl)
            n162 = Divide(x=w211, y=w209) -> (x/y=w210:dbl)
            n163 = Round Toward +Infinity(x=w210) -> (ceil(x): smallest int >= x=w215:dbl)
            n164 = To Long Integer(number=w215) -> (32bit integer=w206:i32)
            n165 = property on="no. of frames" class="DigNum (strict)"(error in=w207, "Val(Sgnl)"=w206) -> (error out=w205:errorcluster)  [unwired: 1 in, 1 out]
          }
          event "x pixels", "y lines", "x aspect", "y aspect", "no. of frames", "no. of averagings", "step": Value Change {
            n166 = event-data() -> ()  [unwired: 2 out]
            n167 = local write "settings enforced?"(FALSE ("settings enforced?")) -> ()
            n168 = call "checkout.vi"("locked by?"="parameter value change", "error in (no error)"=w231) -> ("error out"=w251:errorcluster, "GenericScanMode out"=w250:refnum<class "GenericImagingMode.lvclass">)  [unwired: 8 in]
            n169 = To More Specific Class(target class=w244, reference=w250, error in=w251) -> (specific class reference=w227:refnum<class "ImagingModeDL090130Frame.lvclass">, error out=w223:errorcluster)
            n170 = Unbundle By Name(w227) -> ("SpeedConstant"=w224:T3)
            n171 = case "What is kept constant?" shown="\"pixel dwell time\", Default" w224 {
              tunnel: [w254 w261 w266] -> w228
              tunnel: w227 -> [w256 w260 w264]
              tunnel: [w255 w259 w267] -> w226
              tunnel: w223 -> [w257 w262 w265]
              frame "pixel dwell time", Default {
                n172 = local read "pixel dwell time"() -> (w253:dbl[unit])
                n173 = call-dynamic "set_speed_params.vi"("pixel-dwell time"=w253, "error in (no error)"=w257, "ImagingModeDL090130Frame in"=w256) -> ("error out"=w254:errorcluster, "ImagingModeDL090130Frame out"=w255:refnum<class "ImagingModeDL090130Frame.lvclass">)  [unwired: 7 in]
              }
              frame "line scan time" {
                n174 = local read "line scan time"() -> (w258:dbl[unit])
                n175 = call-dynamic "set_speed_params.vi"("error in (no error)"=w262, "line-scan time"=w258, "ImagingModeDL090130Frame in"=w260) -> ("error out"=w261:errorcluster, "ImagingModeDL090130Frame out"=w259:refnum<class "ImagingModeDL090130Frame.lvclass">)  [unwired: 7 in]
              }
              frame "frame rate" {
                n176 = local read "frame rate"() -> (w263:dbl[unit])
                n177 = call-dynamic "set_speed_params.vi"("error in (no error)"=w265, "frame rate"=w263, "ImagingModeDL090130Frame in"=w264) -> ("error out"=w266:errorcluster, "ImagingModeDL090130Frame out"=w267:refnum<class "ImagingModeDL090130Frame.lvclass">)  [unwired: 7 in]
              }
            }
            n178 = Wait (ms)(milliseconds to wait=u32 500) -> ()  [unwired: 1 out]
            n179 = Bundle By Name(cluster=w226, "ResolutionX"="x pixels", "ResolutionY"="y lines", "AspectRatioX"="x aspect", "AspectRatioY"="y aspect", "AveragingRepetitions"="no. of averagings", "Frames"="no. of frames", "StepSize"="step") -> (w225:refnum<class "ImagingModeDL090130Frame.lvclass">)
            n180 = property on="settings" class="XSettings (strict)"(error in=w228, "Property"=TRUE ("is user-defined?")) -> (error out=w229:errorcluster)  [unwired: 1 in, 1 out]
            n181 = call-dynamic "checkin.vi"("error in (no error)"=w229, "GenericScanMode in"=w225) -> ("error out"=w241:errorcluster, "GenericScanMode out"=w245:refnum<class "ImagingModeDL090130Frame.lvclass">)  [unwired: 8 in]
            n182 = Scan From String(input string="update", error in=w241, default 1=internal_trigger_enum."update" ("internal trigger")) -> (error out=w240:errorcluster, output 1=w239:T4)  [unwired: 2 in, 2 out]
          }
          event Value Change {
            n183 = event-data() -> ("CtlRef"=w277:refnum<vi>)  [unwired: 1 out]
            n184 = property class="Enum (strict)"(reference=w277, error in=w269) -> (error out=w268:errorcluster, "Label.Text"=w276:string)  [unwired: 1 out]
            n185 = call "checkout.vi"("locked by?"=w276, "error in (no error)"=w268) -> ("error out"=w279:errorcluster, "GenericScanMode out"=w278:refnum<class "GenericImagingMode.lvclass">)  [unwired: 8 in]
            n186 = To More Specific Class(target class=w275, reference=w278, error in=w279) -> (specific class reference=w272:refnum<class "ImagingModeDL090130Frame.lvclass">, error out=w274:errorcluster)
            n187 = Bundle By Name(cluster=w272, "SpeedConstant"="keep constant") -> (w270:refnum<class "ImagingModeDL090130Frame.lvclass">)
            n188 = call-dynamic "checkin.vi"("error in (no error)"=w274, "GenericScanMode in"=w270) -> ("error out"=w273:errorcluster)  [unwired: 8 in, 1 out]
          }
          event "settings enforced?": Value Change {
            n189 = event-data() -> ("CtlRef"=w287:refnum<vi>)  [unwired: 1 out]
            n190 = property class="Bool (strict)"(reference=w287, error in=w286) -> (error out=w285:errorcluster, "Label.Text"=w284:string)  [unwired: 1 out]
            n191 = call "checkout.vi"("locked by?"=w284, "error in (no error)"=w285) -> ("error out"=w311:errorcluster, "GenericScanMode out"=w310:refnum<class "GenericImagingMode.lvclass">)  [unwired: 8 in]
            n192 = To More Specific Class(target class=w309, reference=w310, error in=w311) -> (specific class reference=w290:refnum<class "ImagingModeDL090130Frame.lvclass">, error out=w292:errorcluster)
            n193 = local read "XIntensityCompensation"() -> (w298:cluster{"A":dbl, "lambda":dbl[unit], "C":dbl})
            n194 = local read "no. of averagings"() -> (w302:i32)
            n195 = local read "translation mode"() -> (w299:T2)
            n196 = local read "return to origin?"() -> (w300:bool)
            n197 = local read "keep constant"() -> (w282:T3)
            n198 = local read "no. of frames"() -> (w303:i32)
            n199 = local read "x aspect"() -> (w305:dbl)
            n200 = local read "y aspect"() -> (w304:dbl)
            n201 = local read "x pixels"() -> (w307:i32)
            n202 = local read "y lines"() -> (w306:i32)
            n203 = local read "step"() -> (w301:dbl[unit])
            n204 = local read "frame rate"() -> (w288:dbl[unit])
            n205 = call-dynamic "set_speed_params.vi"("error in (no error)"=w292, "frame rate"=w288, "ImagingModeDL090130Frame in"=w290) -> ("error out"=w291:errorcluster, "ImagingModeDL090130Frame out"=w289:refnum<class "ImagingModeDL090130Frame.lvclass">)  [unwired: 7 in]
            n206 = Bundle By Name(cluster=w289, "ResolutionX"=w307, "ResolutionY"=w306, "AspectRatioX"=w305, "AspectRatioY"=w304, "SpeedConstant"=w282, "Frames"=w303, "AveragingRepetitions"=w302, "StepSize"=w301, "ReturnToOrigin"=w300, "TranslationMode"=w299, "IntensityCompensationParameters"=w298) -> (w308:refnum<class "ImagingModeDL090130Frame.lvclass">)
            n207 = call-dynamic "checkin.vi"("error in (no error)"=w291, "GenericScanMode in"=w308) -> ("error out"=w295:errorcluster, "GenericScanMode out"=w283:refnum<class "ImagingModeDL090130Frame.lvclass">)  [unwired: 8 in]
            n208 = Scan From String(input string="update", error in=w295, default 1=internal_trigger_enum."update" ("internal trigger")) -> (error out=w294:errorcluster, output 1=w293:T4)  [unwired: 2 in, 2 out]
          }
          event Value Change {
            n209 = event-data() -> ("CtlRef"=w321:refnum<vi>)  [unwired: 1 out]
            n210 = property class="Enum (strict)"(reference=w321, error in=w320) -> (error out=w323:errorcluster, "Label.Text"=w322:string)  [unwired: 1 out]
            n211 = call "checkout.vi"("locked by?"=w322, "error in (no error)"=w323) -> ("error out"=w328:errorcluster, "GenericScanMode out"=w327:refnum<class "GenericImagingMode.lvclass">)  [unwired: 8 in]
            n212 = To More Specific Class(target class=w318, reference=w327, error in=w328) -> (specific class reference=w325:refnum<class "ImagingModeDL090130Frame.lvclass">, error out=w326:errorcluster)
            n213 = Bundle By Name(cluster=w325, "TranslationMode"="translation mode") -> (w324:refnum<class "ImagingModeDL090130Frame.lvclass">)
            n214 = call-dynamic "checkin.vi"("error in (no error)"=w326, "GenericScanMode in"=w324) -> ("error out"=w315:errorcluster, "GenericScanMode out"=w319:refnum<class "ImagingModeDL090130Frame.lvclass">)  [unwired: 8 in]
            n215 = property on="settings" class="XSettings (strict)"(error in=w315, "Property"=TRUE ("is user-defined?")) -> (error out=w314:errorcluster)  [unwired: 1 in, 1 out]
          }
          event Value Change {
            n216 = event-data() -> ()  [unwired: 2 out]
            n217 = Current VI's Path() -> (path=w333:path)
            n218 = call-dynamic "undock.vi"("error in (no error)"=w336, "undock?"="button:undock", "VI path"=w333, "component in"=w332) -> ("error out"=w335:errorcluster, "component out"=w331:refnum<class "ImagingModeDL090130Frame.lvclass">)  [unwired: 6 in]
          }
          event "XIntensityCompensation": Value Change {
            n219 = event-data() -> ("CtlRef"=w350:refnum<vi>)  [unwired: 1 out]
            n220 = property class="XIntensityCompensation (strict)"(reference=w350, error in=w342) -> (error out=w341:errorcluster, "Label.Text"=w347:string)  [unwired: 1 out]
            n221 = call "checkout.vi"("locked by?"=w347, "error in (no error)"=w341) -> ("error out"=w349:errorcluster, "GenericScanMode out"=w351:refnum<class "GenericImagingMode.lvclass">)  [unwired: 8 in]
            n222 = To More Specific Class(target class=w344, reference=w351, error in=w349) -> (specific class reference=w340:refnum<class "ImagingModeDL090130Frame.lvclass">, error out=w343:errorcluster)
            n223 = Bundle By Name(cluster=w340, "IntensityCompensationParameters"="XIntensityCompensation") -> (w346:refnum<class "ImagingModeDL090130Frame.lvclass">)
            n224 = call-dynamic "checkin.vi"("error in (no error)"=w343, "GenericScanMode in"=w346) -> ("error out"=w348:errorcluster, "GenericScanMode out"=w345:refnum<class "ImagingModeDL090130Frame.lvclass">)  [unwired: 8 in]
          }
          event "finished?": Value Change {
            n225 = event-data() -> ()  [unwired: 2 out]
          }
        }
        n226 = Unbundle By Name(w68) -> ("status"=w71:bool)
        n227 = To More Generic Class(target class=refnum<class "GenericComponent.lvclass"> refnum ("GenericComponent.lvclass"), reference=w59) -> (generic class reference=w62:refnum<class "GenericComponent.lvclass">)
        n228 = local write "settings"(w62) -> ()
        n229 = Or(x=w71, y=w70) -> (x .or. y?=w69:bool)
        n230 = To Variant(anything=w64) -> (Variant=w66:variant)
        n231 = call-dynamic "send_generic_trigger.vi"("error in (no error)"=w68, "trigger type"=trigger_type_enum."internal", "trigger variant"=w66, "GenericToplevelComponent in"=w59) -> ("error out"=w67:errorcluster, "GenericToplevelComponent out"=w60:refnum<class "ImagingModeDL090130Frame.lvclass">)  [unwired: 4 in, 2 out]
        "event error" <- w67
        "event handling loop counter" <- w74
      }
      n232 = call-dynamic "flush_trigger_queue.vi"("error in (no error)"=w35, "GenericToplevelComponent in"=w30) -> ("error out"=w34:errorcluster)  [unwired: 8 in, 1 out]
      n233 = property on="finished?" class="Bool (strict)"(error in=w56, "Val(Sgnl)"=w36) -> (error out=w50:errorcluster)  [unwired: 1 in, 1 out]
      n234 = call "send_error.vi"("additional message"="Error after event loop...", "error in (no error)"=w34) -> ("error out"=w44:errorcluster)  [unwired: 9 in]
      n235 = call "send_error.vi"("additional message"="Error after statemachine loop...", "error in (no error)"=w50) -> ("error out"=w48:errorcluster)  [unwired: 9 in]
      n236 = Merge Errors(w44, w48) -> (w46:errorcluster)
      n237 = call "checkout.vi"("locked by?"="", "error in (no error)"=w46) -> ("error out"=w45:errorcluster)  [unwired: 8 in, 1 out]
    }
    frame Error {
    }
  }
  "error out" <- w26
  "ImagingModeDL090130Frame out" <- w25
